vi "Build Mappings Array.vi"(6 "VI Names":string[](array[string]), 8 "error in (no error)":errorcluster, 9 "RESTful VI routing template":T1={"Template"="", "Routing Type"=enum."Static", "HTTP Method Type"=enum."GET", "VIName"="", "Default String"="", "Require API key"=FALSE, "Auth permissions"=[], "eng_Static Alias"="", "Required Privilege"=""}, 10 "Controls and Indicators for XML":T5(array[cluster]), 11 "Description in":T6) -> (0 "error out":errorcluster, 3 "Description out":T6)   [LabVIEW 2020, in "Web Service Description.lvlib"]
uses:
  <vilib>/AppBuilder/Engine/WebServiceDescription/Web Service Description.lvlib
  <vilib>/AppBuilder/Engine/WebServiceDescription/LVDataTypes/LVType/LVType.lvclass
  <vilib>/AppBuilder/Engine/WebServiceDescription/Terminal Info.ctl
  <vilib>/AppBuilder/Engine/WebServiceDescription/URL Mapping Info.ctl
  <vilib>/AppBuilder/AB_Classes/RESTful/AB_RESTful_HTTPMethodType.ctl
  <vilib>/AppBuilder/Engine/WebServiceDescription/Response.ctl
  <vilib>/AppBuilder/Engine/WebServiceDescription/Web Service Description Info.ctl
  <vilib>/AppBuilder/AB_Classes/Source/RESTfulVI/Configure_RESTfulVI/AB_RESTful_OutputType.ctl
  <vilib>/AppBuilder/AB_Classes/Source/RESTfulVI/Configure_RESTfulVI/AB_RESTful_OutputFormat.ctl
  <vilib>/AppBuilder/AB_Classes/RESTful/AB_RESTful_RoutingType.ctl
  <vilib>/AppBuilder/AB_Classes/RESTful/AB_RESTful_RoutingTemplate.ctl
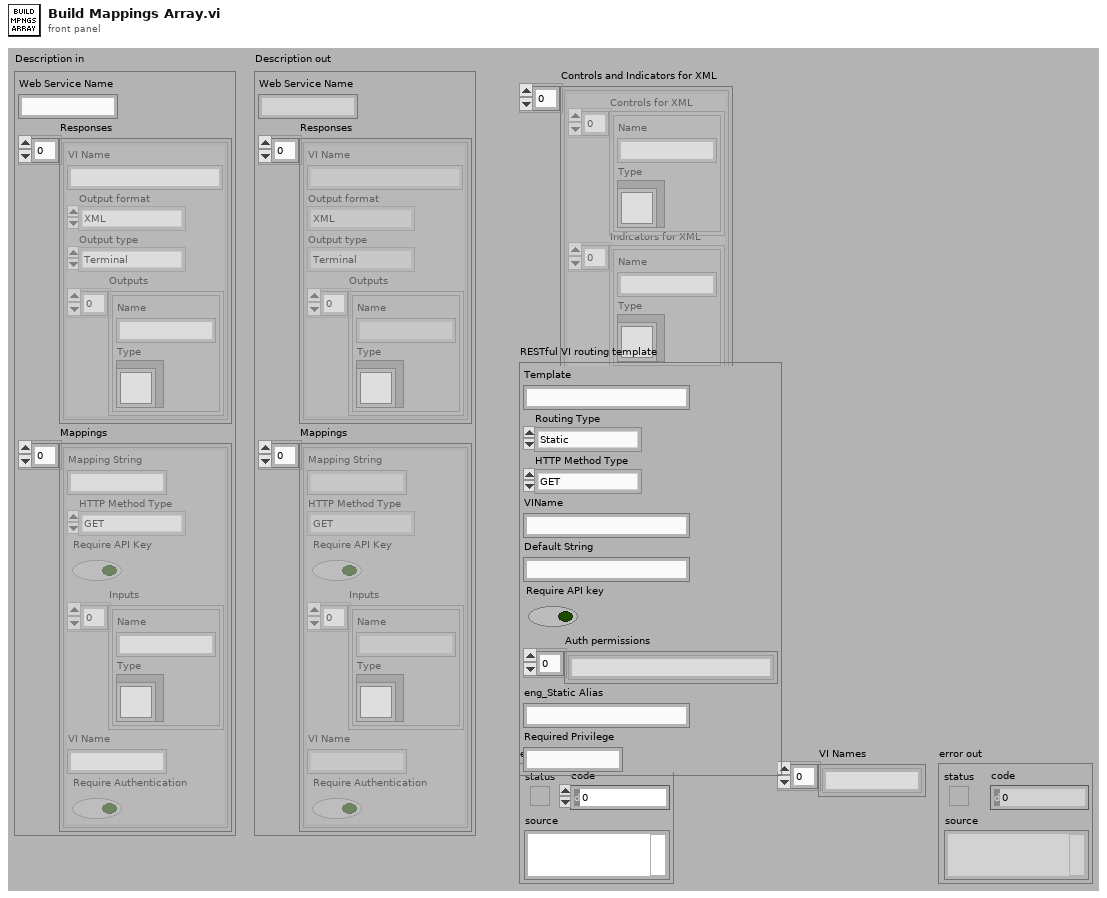
[diagram p1: front panel]
types:
  T1 = typedef "AB_RESTful_RoutingTemplate.ctl" = cluster{"Template":string, "Routing Type":T2, "HTTP Method Type":T3, "VIName":string, "Default String":string, "Require API key":bool, "Auth permissions":string[], "eng_Static Alias":string, "Required Privilege":string}
  T2 = typedef "AB_RESTful_RoutingType.ctl" = enum32{"Method", "Static"}
  T3 = typedef "AB_RESTful_HTTPMethodType.ctl" = enum32{"GET", "POST", "PUT", "DELETE"}
  T4 = typedef "Web Service Description.lvlib/Terminal Info.ctl" = cluster{"Name":string, "Type":refnum<class "LVType.lvclass">}
  T5 = cluster{"Controls for XML":T4[], "Indicators for XML":T4[]}[]
  T6 = typedef "Web Service Description.lvlib/Web Service Description Info.ctl" = cluster{"Web Service Name":string, "Responses":T7[], "Mappings":T10[]}
  T7 = typedef "Web Service Description.lvlib/Response.ctl" = cluster{"VI Name":string, "Output format":T8, "Output type":T9, "Outputs":T4[]}
  T8 = typedef "AB_RESTful_OutputFormat.ctl" = enum32{"XML", "Text", "HTML", "JSON"}
  T9 = typedef "AB_RESTful_OutputType.ctl" = enum32{"Terminal", "Stream"}
  T10 = typedef "Web Service Description.lvlib/URL Mapping Info.ctl" = cluster{"Mapping String":string, "HTTP Method Type":T3, "Require API Key":bool, "Inputs":T4[], "VI Name":string, "Require Authentication":bool}
  T11 = cluster{"Controls for XML":T4[], "Indicators for XML":T4[]}
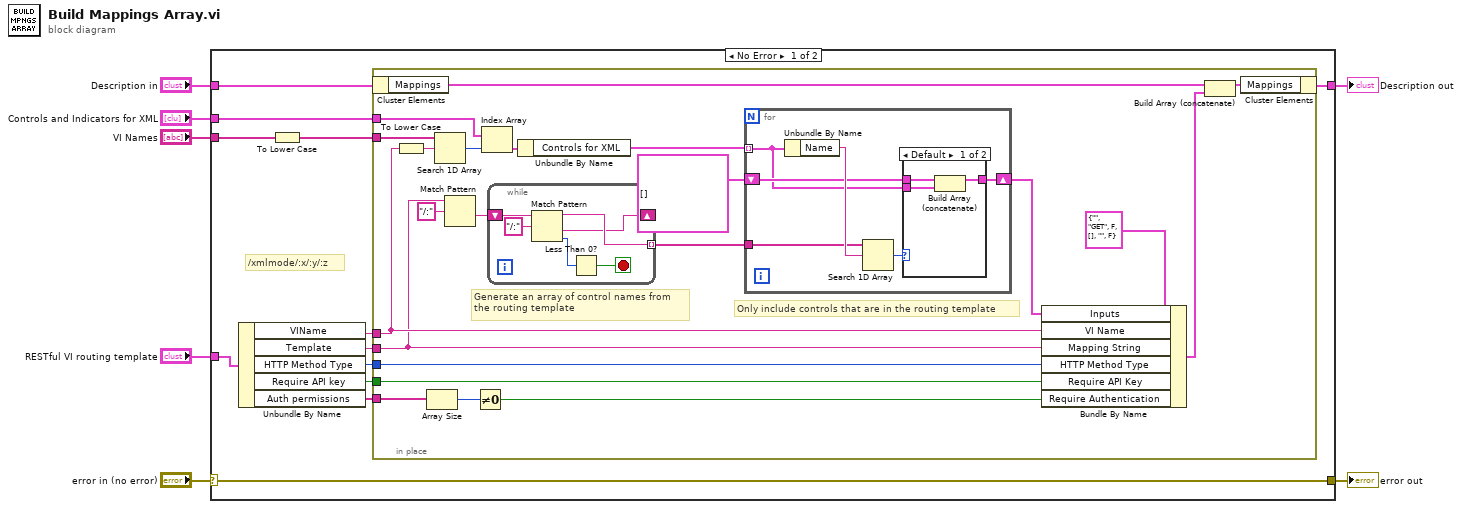
[diagram p0: block diagram]
diagram:
  n1 = case shown="No Error" "error in (no error)" {
    selector: "error in (no error)" -> [w16 w59]
    tunnel: [w16 w59] -> w6
    tunnel: "Description in" -> [w19 w58]
    tunnel: [w18 w58] -> w4
    tunnel: "VI Names" -> [w17 _]
    tunnel: "RESTful VI routing template" -> [w15 _]
    tunnel: "Controls and Indicators for XML" -> [w10 _]
    frame No Error {
      # "/xmlmode/:x/:y/:z"
      n2 = Unbundle By Name(w15) -> ("VIName"=w14:string, "Template"=w13:string, "HTTP Method Type"=w12:T3, "Require API key"=w11:bool, "Auth permissions"=w8:string[])
      n3 = To Lower Case(string=w17) -> (all lower case string=w9:string[])
      n4 = in-place {
        in-place-border: w9 -> [w34]
        in-place-border: w14 -> [w35]
        in-place-border: w13 -> [w25]
        in-place-border: w12 -> [w37]
        in-place-border: w11 -> [w36]
        in-place-border: w10 -> [w31]
        in-place-border: w8 -> [w22]
        # "Generate an array of control names from\nthe routing template"
        # "Only include controls that are in the routing template"
        n5 = in-place-cluster #1(w19) -> ("Mappings"=w40:T10[])
        n6 = To Lower Case(string=w35) -> (all lower case string=w33:string)
        n7 = Array Size(array=w22) -> (size(s)=w21:i32)
        n8 = Search 1D Array(1D array=w34, element=w33) -> (index of element=w32:i32)  [unwired: 1 in]
        n9 = Match Pattern(string=w25, regular expression="/:") -> (after substring=w24:string)  [unwired: 1 in, 3 out]
        n10 = Not Equal To 0?(x=w21) -> (x != 0?=w20:bool)
        n11 = Index Array(array=w31, index=w32) -> (element=w30:T11)
        n12 = while {
          shift-right: [w54] -> _
          shift-left: w24 -> [w56]
          tunnel: [w55] -> w23 mode=indexing
          stop <- w52 stop-if-true
          n13 = Match Pattern(string=w56, regular expression="/:") -> (before substring=w55:string, after substring=w54:string, offset past match=w53:i32)  [unwired: 1 in, 1 out]
          n14 = Less Than 0?(x=w53) -> (x < 0?=w52:bool)
        }
        n15 = Unbundle By Name(w30) -> ("Controls for XML"=w29:T4[])
        n16 = for {
          tunnel: w29 -> [w43] mode=indexing
          shift-right: [w44] -> w27
          shift-left: T4[] [] ("Controls for XML") -> [w45]
          tunnel: w23 -> [w42]
          n17 = Unbundle By Name(w43) -> ("Name"=w47:string)
          n18 = Search 1D Array(1D array=w42, element=w47) -> (index of element=w46:i32)  [unwired: 1 in]
          n19 = case shown="Default" w46 {
            tunnel: w45 -> [w50 w51]
            tunnel: [w49 w51] -> w44
            tunnel: w43 -> [w48 _]
            frame Default {
              n20 = Build Array (concatenate)(w50, w48) -> (w49:T4[])
            }
            frame -1 {
            }
          }
        }
        n21 = Bundle By Name(cluster=T10 {"Mapping String"="", "HTTP Method Type"=enum."GET", "Require API Key"=FALSE, "Inputs"=[], "VI Name"="", "Require Authentication"=FALSE} ("URL Mapping"), "Inputs"=w27, "VI Name"=w35, "Mapping String"=w25, "HTTP Method Type"=w37, "Require API Key"=w36, "Require Authentication"=w20) -> (w38:T10)
        n22 = Build Array (concatenate)(w40, w38) -> (w39:T10[])
        n23 = in-place-cluster #1("Mappings"=w39) -> (w18:T6)
      }
    }
    frame Error {
    }
  }
  "error out" <- w6
  "Description out" <- w4
